vi "Find COM device.vi"(9 "Serial configs":T1={"Baud Rate"=57600, "Data Bits"=7, "Parity"=1, "Stop Bits"=10, "Flow Control"=0, "Termination Character"=10, "Enable Term Character"=FALSE} {"Termination Character" format="%x" items=["NUL 0x00"=0, "TAB 0x09"=9, "LF 0x0A"=10, "CR 0x0D"=13, "ESC 0x1B"=27]; "Flow Control" items=["None", "XON/XOFF", "RTS/CTS", "XON/XOFF & RTS/CTS", "DTR/DSR", "XON/XOFF & DTR/DSR"]; "Stop Bits" items=["1.0"=10, "1.5"=15, "2.0"=20]; "Parity" items=["None", "Odd", "Even", "Mark", "Space"]; "Data Bits" items=["7"=7, "8"=8]; "Baud Rate" items=["300"=300, "600"=600, "1200"=1200, "2400"=2400, "4800"=4800, "9600"=9600, "19200"=19200, "38400"=38400, "57600"=57600]}, 10 "ID string":string, 11 "IDN cmd":string="*IDN?") -> (2 "IDN responses":string[](array[string]), 3 "VISA refs":refnum<visa-resource-name>[](array[refnum]))   [LabVIEW 2021, in "MatS Libs.lvlib"]
doc: "Searches for uninitialized instruments connected to a serial (COM) port. It seraches for match with <B>match string</B> in response to <B>IDN cmd</B> (for devices that comply with IEEE-488 it is *IDN?).\nEmpty array is returned if no device match."
uses:
  d722f5fc-b54c-40b4-a879-b91740defc9d.vi
  <userlib>/MatS Libs/MatS Libs.lvlib
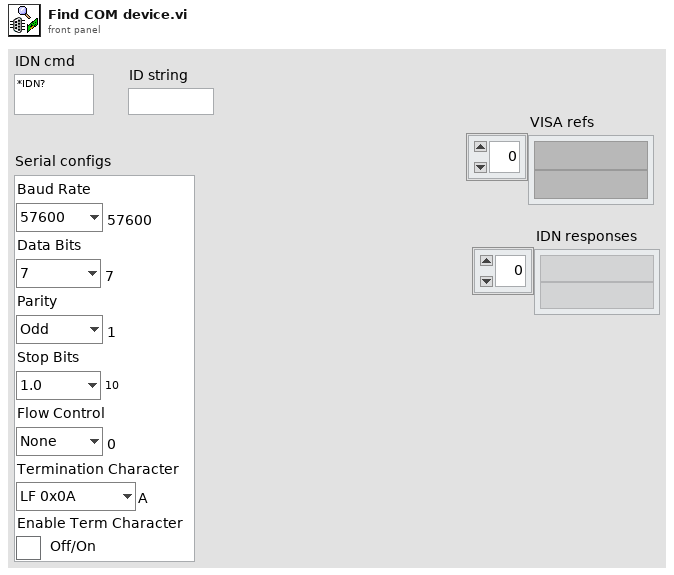
[diagram p1: front panel]
types:
  T1 = cluster{"Baud Rate":u32, "Data Bits":u16, "Parity":u16, "Stop Bits":u16, "Flow Control":u16, "Termination Character":u8, "Enable Term Character":bool}
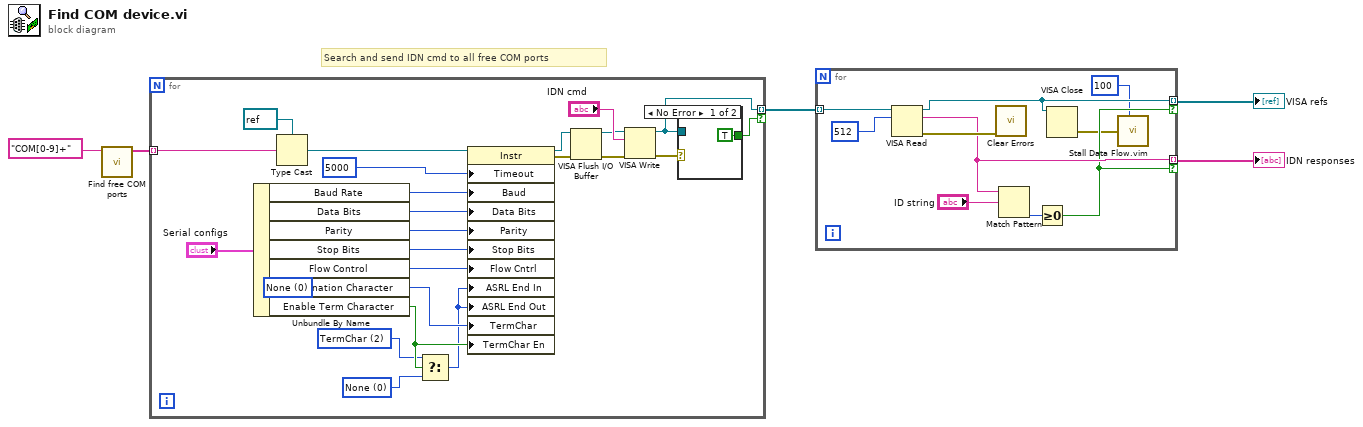
[diagram p0: block diagram]
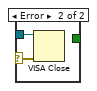
[diagram p2: hidden frame]
diagram:
  # "Search and send IDN cmd to all free COM ports"
  n1 = call <userlib>:"Find free COM ports.vi"("regular expression"="COM[0-9]+") -> ("Free COM ports"=w5:string[])  [unwired: 10 in]
  n2 = for {
    tunnel: w5 -> [w20] mode=indexing
    tunnel: [w24] -> w4 mode=indexing if=w23
    w11 = u16 2 items=["None", "Last Bit", "TermChar", "Break"] ("Serial Settings:End Mode for Writes")
    w10 = u16 0 items=["None", "Last Bit", "TermChar", "Break"] ("Serial Settings:End Mode for Writes")
    (unwired) u16 0 items=["None", "Odd", "Even", "Mark", "Space"] ("Serial Settings:Parity")
    n3 = Unbundle By Name("Serial configs") -> ("Baud Rate"=w15:u32, "Data Bits"=w14:u16, "Parity"=w13:u16, "Stop Bits"=w17:u16, "Flow Control"=w18:u16, "Termination Character"=w19:u8, "Enable Term Character"=w12:bool)
    n4 = Type Cast(type=refnum<visa-resource-name> refnum ("PSU COM"), x=w20) -> (*(type *) &x=w21:refnum<visa-resource-name>)
    n5 = Select(t=w11, s=w12, f=w10) -> (s? t:f=w9:u16)
    n6 = property class="Instr"(reference=w21, "Timeout"=u32 5000 ("General Settings:Timeout Value"), "Baud"=w15, "Data Bits"=w14, "Parity"=w13, "Stop Bits"=w17, "Flow Cntrl"=w18, "ASRL End In"=w9, "ASRL End Out"=w9, "TermChar"=w19, "TermChar En"=w12) -> (reference out=w7:refnum<visa-resource-name>, error out=w8:errorcluster)  [unwired: 1 in]
    n7 = VISA Flush I/O Buffer(VISA resource name=w7, error in (no error)=w8) -> (VISA resource name out=w27:refnum<visa-resource-name>, error out=w26:errorcluster)  [unwired: 1 in]
    n8 = VISA Write(VISA resource name=w27, write buffer="IDN cmd", error in (no error)=w26) -> (VISA resource name out=w24:refnum<visa-resource-name>, error out=w25:errorcluster)  [unwired: 1 out]
    n9 = case shown="No Error" w25 {
      selector: w25 -> [_ w31]
      tunnel: w24 -> [_ w30]
      tunnel: [TRUE _] -> w23
      frame No Error {
      }
      frame Error {
        n10 = VISA Close(VISA resource name=w30, error in (no error)=w31) -> ()  [unwired: 1 out]
      }
    }
  }
  n11 = for {
    tunnel: w4 -> [w41] mode=indexing
    tunnel: [w34] -> w3 mode=indexing if=w35
    tunnel: [w36] -> w2 mode=indexing if=w35
    n12 = VISA Read(VISA resource name=w41, byte count=u32 512) -> (VISA resource name out=w34:refnum<visa-resource-name>, read buffer=w36:string, error out=w37:errorcluster)  [unwired: 1 in, 1 out]
    n13 = call <vilib>:"Clear Errors.vi"("error in (no error)"=w37) -> ()  [unwired: 5 in, 2 out]
    n14 = Match Pattern(string=w36, regular expression="ID string") -> (offset past match=w38:i32)  [unwired: 1 in, 3 out]
    n15 = Greater Or Equal To 0?(x=w38) -> (x >= 0?=w35:bool)
    n16 = VISA Close(VISA resource name=w34) -> (error out=w33:errorcluster)  [unwired: 1 in]
    n17 = call "Stall Data Flow.vim"("value in"=w33, "milliseconds to wait"=u32 100) -> ()  [unwired: 2 out]
  }
  "VISA refs" <- w3
  "IDN responses" <- w2
